vi "split_readouts.vi"(8 "repetitions":i32 caption="Repetitions", 9 "read_width_us":dbl, 10 "pulse_period_us":dbl, 11 "timetags":u32[](array[numeric])) -> (2 "q_photons":i32[](array[numeric]), 3 "readouts":u32[][](array[numeric]))   [LabVIEW 2014]
panel:
  out "Waveform Chart 4":u32[][](graph)
  out "limits_period":dbl[](array[numeric])
  out "limits_read":dbl[](array[numeric])
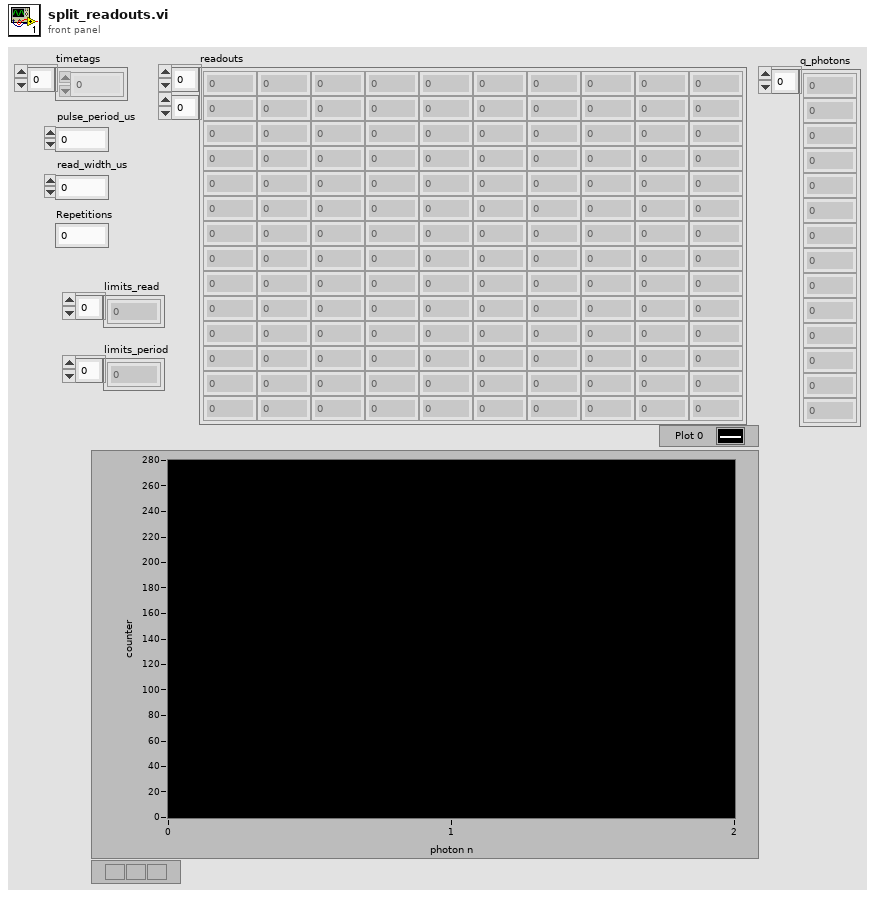
[diagram p1: front panel]
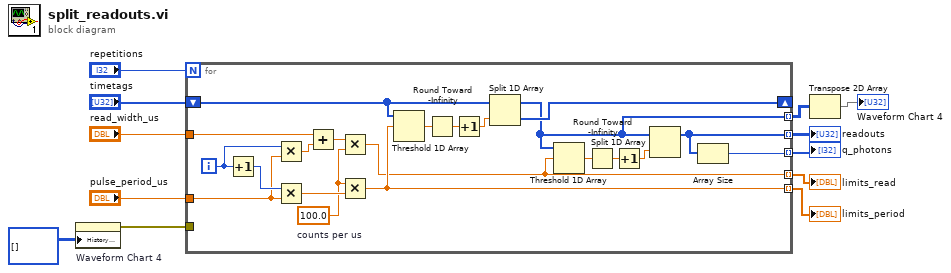
[diagram p0: block diagram]
diagram:
  n1 = property on="Waveform Chart 4" class="WFChart (strict)"("History Data"=u32[][] []) -> (error out=w3:errorcluster)  [unwired: 2 in, 1 out]
  n2 = for {
    N: "repetitions" -> [_]
    shift-right: [w20] -> _
    shift-left: "timetags" -> [w22]
    tunnel: "pulse_period_us" -> [w30]
    tunnel: "read_width_us" -> [w28]
    tunnel: [w21] -> w8 mode=indexing
    tunnel: [w16] -> w9 mode=indexing
    tunnel: [w14] -> w7 mode=indexing
    tunnel: [w15] -> w6 mode=indexing
    tunnel: w3 -> [_]
    tunnel: [w13] -> w2 mode=indexing
    i -> [w31]
    w26 = 100.0  # counts per us
    n3 = Increment(x=w31) -> (x+1=w32:i32)
    n4 = Multiply(x=w31, y=w30) -> (x*y=w27:dbl)
    n5 = Multiply(x=w32, y=w30) -> (x*y=w33:dbl)
    n6 = Add(x=w28, y=w27) -> (x+y=w29:dbl)
    n7 = Multiply(x=w29, y=w26) -> (x*y=w16:dbl)
    n8 = Multiply(x=w26, y=w33) -> (x*y=w21:dbl)
    n9 = Threshold 1D Array(2:w21, 3:w22) -> (0:w23:dbl)  [unwired: 1 in]
    n10 = Round Toward -Infinity(1:w23) -> (0:w24:dbl)
    n11 = Increment(x=w24) -> (x+1=w25:dbl)
    n12 = Split 1D Array(array=w22, index=w25) -> (first subarray=w15:u32[], second subarray=w20:u32[])
    n13 = Threshold 1D Array(2:w16, 3:w15) -> (0:w19:dbl)  [unwired: 1 in]
    n14 = Round Toward -Infinity(1:w19) -> (0:w18:dbl)
    n15 = Increment(x=w18) -> (x+1=w17:dbl)
    n16 = Split 1D Array(array=w15, index=w17) -> (first subarray=w14:u32[])  [unwired: 1 out]
    n17 = Array Size(array=w14) -> (size(s)=w13:i32)
  }
  "readouts" <- w7
  "limits_read" <- w9
  "limits_period" <- w8
  "q_photons" <- w2
  n18 = Transpose 2D Array(2D array=w6) -> (transposed array=→"Waveform Chart 4":u32[][])
